vi "HoldPosition.vi"(10 "Pot Value":dbl, 11 "Joystick":bool[](array[boolean])) -> (2 "Setpoint Value":dbl, 3 "Force Value":i32)   [LabVIEW 2014]
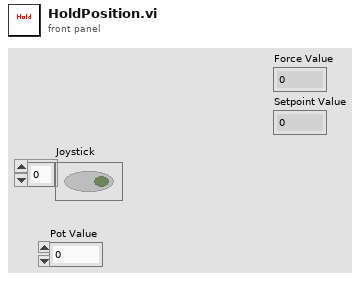
[diagram p1: front panel]
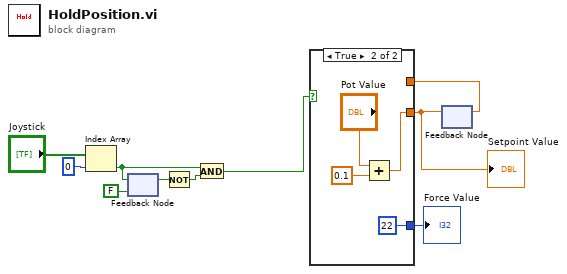
[diagram p0: block diagram]
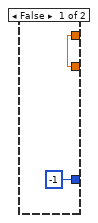
[diagram p2: hidden frame]
diagram:
  n1 = Index Array(array="Joystick", index=0) -> (element=w6:bool)
  n2 = feedback-in #1(w6) -> ()
  n3 = feedback #1(FALSE ("Boolean")) -> (w8:bool)
  n4 = Not(x=w8) -> (.not. x?=w7:bool)
  n5 = And(x=w6, y=w7) -> (x .and. y?=w4:bool)
  n6 = feedback #2() -> (w2:dbl)  [unwired: 1 in]
  n7 = case shown="True" w4 {
    tunnel: [w12 w14] -> w3
    tunnel: w2 -> [w12 _]
    tunnel: [-1 22] -> w1
    frame False {
    }
    frame True {
      n8 = Add(x="Pot Value", y=0.1) -> (x+y=w14:dbl)
    }
  }
  "Force Value" <- w1
  "Setpoint Value" <- w3
  n9 = feedback-in #2(w3) -> ()
